vi "For and while loop.vi"() -> ()   [LabVIEW 2020]
panel:
  out "current time":timestamp
  out "Sum of N numbers using While loop":i32
  out "Sum of N numbers using For loop":i32
  in  "Input":i32
  in  "Input":i32
  # "2-a)"
  # "2-b)"
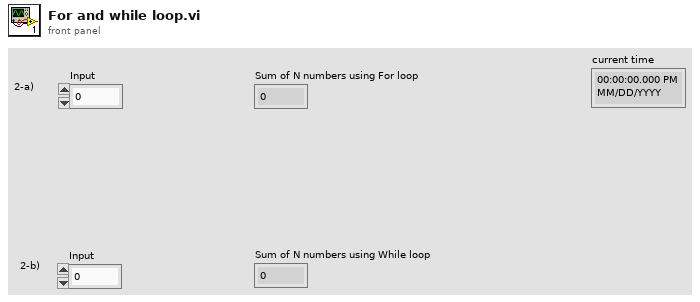
[diagram p1: front panel]
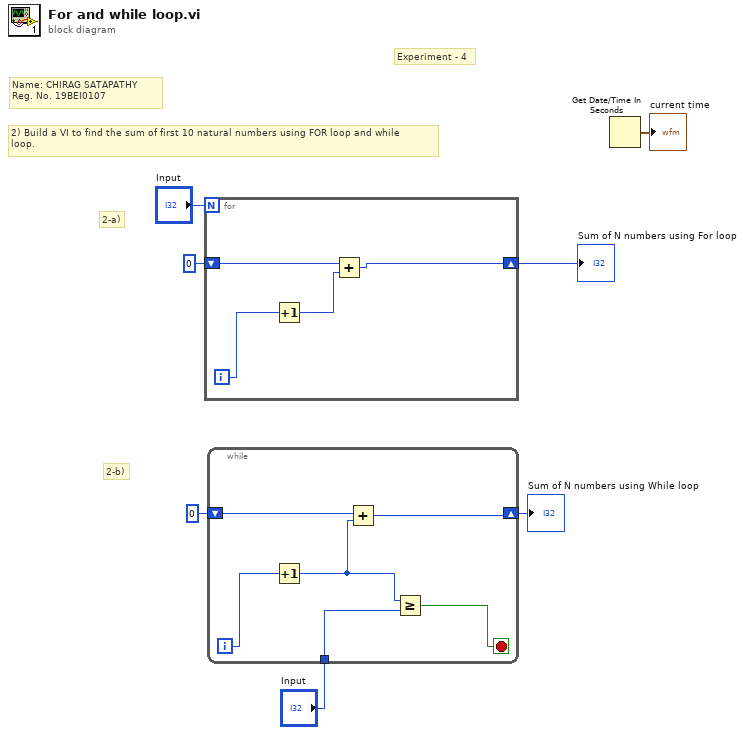
[diagram p0: block diagram]
diagram:
  # "Name: CHIRAG SATAPATHY\nReg. No. 19BEI0107"
  # "2-b)"
  # "2-a)"
  # "Experiment - 4"
  # "2) Build a VI to find the sum of first 10 natural numbers using FOR loop and while\nloop."
  n1 = for {
    N: "Input" -> [_]
    shift-right: [w8] -> w5
    shift-left: 0 -> [w9]
    i -> [w11]
    n2 = Increment(x=w11) -> (x+1=w10:i32)
    n3 = Add(x=w9, y=w10) -> (x+y=w8:i32)
  }
  "Sum of N numbers using For loop" <- w5
  n4 = while {
    tunnel: "Input" -> [w15]
    shift-right: [w13] -> w3
    shift-left: 0 -> [w12]
    i -> [w17]
    stop <- w14 stop-if-true
    n5 = Increment(x=w17) -> (x+1=w16:i32)
    n6 = Add(x=w12, y=w16) -> (x+y=w13:i32)
    n7 = Greater Or Equal?(x=w16, y=w15) -> (x >= y?=w14:bool)
  }
  "Sum of N numbers using While loop" <- w3
  n8 = Get Date/Time In Seconds() -> (seconds since 1Jan1904=→"current time":timestamp)
